vi "Test Work Dispatcher Broadcast When Dispatching.vi"(8 "error in (no error)":errorcluster, 11 "Work Dispatcher Test in":refnum<class "Work Dispatcher Test.lvclass">) -> (0 "error out":errorcluster, 3 "Work Dispatcher Test out":refnum<class "Work Dispatcher Test.lvclass">)   [LabVIEW 2020, in "Work Dispatcher Test.lvclass"]
uses:
  Work Dispatcher Test.lvclass
  C:/Program Files (x86)/National Instruments/LabVIEW 2020/vi.lib/Asteme/LUnit/Test Case.lvclass
  Processes/Work Dispatcher/Work Dispatcher.lvclass
  C:/Program Files (x86)/National Instruments/LabVIEW 2020/vi.lib/Asteme/Triarc Framework/Process/Process.lvclass
  <vilib>/Asteme/Triarc Framework/Process/Process.lvclass/Process.ctl
  <vilib>/Asteme/LUnit/Test Case.lvclass/Test Case.ctl
  <vilib>/Asteme/LUnit/LUnit Assertion Result.lvclass/LUnit Assertion Result.ctl
  <vilib>/Asteme/Triarc Framework/Broadcast Event Helpers/Execution timer.vi
  <vilib>/Asteme/Triarc Framework/Process/Private/SubVIs/Wait for finish.vi
  <vilib>/Asteme/Triarc Framework/Process/Protected/Messaging/Enqueue Message.vi
  <vilib>/Asteme/Triarc Framework/Process/Private/SubVIs/Set Lifecycle State.vi
  <vilib>/Asteme/Triarc Framework/Process/Public/Lifecycle/Get Lifecycle State.vi
  <vilib>/Asteme/LUnit/Palette/Pass If.vi
  <vilib>/Asteme/LUnit/Set Assertion Type.vi
  <vilib>/Utility/error.llb/Clear Errors.vi
  <vilib>/Asteme/LUnit/Palette/Fail.vi
  <vilib>/Asteme/LUnit/Palette/Pass.vi
  <vilib>/Asteme/LUnit/LUnit Write Assertion Type.vi
  <vilib>/Asteme/LUnit/Add test result.vi
  <vilib>/Asteme/LUnit/LUnit Write Passed.vi
  <vilib>/Asteme/LUnit/LUnit Get Test Case.vi
  <vilib>/Asteme/LUnit/Assertion Result/LUnit Get Test Name.vi
  <vilib>/Asteme/LUnit/LUnit Write Message.vi
  <vilib>/Asteme/LUnit/LUnit Write Description.vi
  <vilib>/Asteme/LUnit/Read Test Case Name.vi
  <vilib>/Asteme/Triarc Framework/Broadcast Event Helpers/Dequeue Broadcast Message.vi
  <vilib>/Utility/error.llb/Error Cluster From Error Code.vi
  <vilib>/Asteme/LUnit/LUnit Assertion Result.lvclass
  <vilib>/Asteme/Triarc Framework/Process/Process.lvclass
  <vilib>/Asteme/LUnit/Test Case.lvclass
  <vilib>/Asteme/Triarc Framework/Broadcast Event Helpers/Broadcast Event Helpers.lvlib
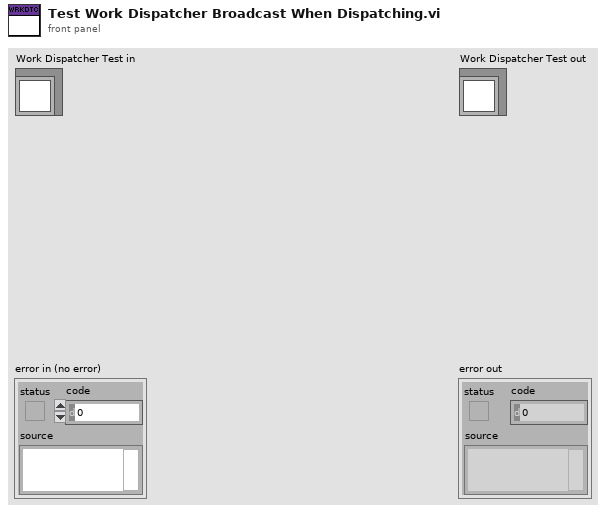
[diagram p1: front panel]
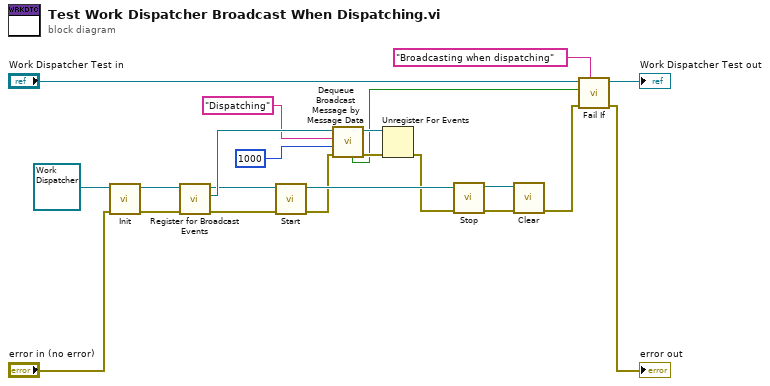
[diagram p0: block diagram]
diagram:
  n1 = call-dynamic "Init.vi"("error in (no error)"="error in (no error)", "Process In"=refnum<class "Work Dispatcher.lvclass"> refnum ("Work Dispatcher.lvclass")) -> ("error out"=w19:errorcluster, "Process Out"=w20:refnum<class "Work Dispatcher.lvclass">)  [unwired: 8 in]
  n2 = call <vilib>:"Register for Broadcast Events.vi"("error in (no error)"=w19, "Process In"=w20) -> ("error out"=w7:errorcluster, "Event Registration Refnum Out"=w15:refnum<event-registration>, "Process Out"=w8:refnum<class "Work Dispatcher.lvclass">)  [unwired: 7 in]
  n3 = call <vilib>:"Start.vi"("error in (no error)"=w7, "Process In"=w8) -> ("error out"=w12:errorcluster, "Process Out"=w18:refnum<class "Work Dispatcher.lvclass">)  [unwired: 8 in]
  n4 = call <vilib>:"Dequeue Broadcast Message by Message Data.vi"("error in (no error)"=w12, "Timeout (-1)"=1000, "Message Data"="Dispatching", "Event Registration Refnum"=w15) -> ("error out"=w11:errorcluster, "Event Registration Refnum Out"=w9:refnum<event-registration>, "Timed Out?"=w1:bool)  [unwired: 3 in, 2 out]
  n5 = Unregister For Events(event registration refnum=w9, error in=w11) -> (error out=w10:errorcluster)
  n6 = call <vilib>:"Stop.vi"("error in (no error)"=w10, "Process In"=w18) -> ("error out"=w16:errorcluster, "Process Out"=w17:refnum<class "Work Dispatcher.lvclass">)  [unwired: 7 in, 1 out]
  n7 = call-dynamic "Clear.vi"("error in (no error)"=w16, "Process In"=w17) -> ("error out"=w2:errorcluster)  [unwired: 9 in]
  n8 = call <vilib>:"Fail If.vi"("Description"="Broadcasting when dispatching", "error in (no error)"=w2, "Fail?"=w1, "Test Case In"="Work Dispatcher Test in") -> ("error out"=→"error out":errorcluster, "Test Case Out"=→"Work Dispatcher Test out":refnum<class "Work Dispatcher Test.lvclass">)  [unwired: 6 in]
